vi "Initialize Hardware References.vi"(8 "error in (no error)":errorcluster, 11 "Hardware Resources in":T1={"DAQmx Channel 1"="", "DAQmx Channel 2"="", "DAQmx Channel 3"="", "Channel 1 Name"="Battery Voltage", "Channel 2 Name"="Battery Current", "Channel 3 Name"="Brake torque", "Input Config Channel 1"=-1, "Input Config Channel 2"=-1, "Input Config Channel 3"=-1, "Offset Channel 1"=0.0, "Offset Channel 2"=0.0, "Offset Channel 3"=0.0, "Scale Channel 1"=0.0, "Scale Channel 2"=0.0, "Scale Channel 3"=0.0, "Sample time"=50, "Samples per second"=1000.0, "Sample mode"=0, "Samples per channel"=0, "DAQmx AI Task"="", "DAQmx Channel 4"="", "Channel 3 Name 2"="", "Input Config Channel 4"=-1, "Offset Channel 4"=0.0, "Scale Channel 4"=0.0} {"Input Config Channel 4" items=["Default"=-1, "RSE"=10083, "NRSE"=10078, "Differential"=10106, "Pseudodifferential"=12529]; "Input Config Channel 3" items=["Default"=-1, "RSE"=10083, "NRSE"=10078, "Differential"=10106, "Pseudodifferential"=12529]; "Input Config Channel 2" items=["Default"=-1, "RSE"=10083, "NRSE"=10078, "Differential"=10106, "Pseudodifferential"=12529]; "Input Config Channel 1" items=["Default"=-1, "RSE"=10083, "NRSE"=10078, "Differential"=10106, "Pseudodifferential"=12529]; "Sample mode" items=["Hardware Timed Single Point"=12522, "Finite Samples"=10178, "Continuous Samples"=10123]}) -> (0 "error out":errorcluster, 3 "Hardware Resources out":T1={"DAQmx Channel 1"="", "DAQmx Channel 2"="", "DAQmx Channel 3"="", "Channel 1 Name"="Battery Voltage", "Channel 2 Name"="Battery Current", "Channel 3 Name"="Brake torque", "Input Config Channel 1"=-1, "Input Config Channel 2"=-1, "Input Config Channel 3"=-1, "Offset Channel 1"=0.0, "Offset Channel 2"=0.0, "Offset Channel 3"=0.0, "Scale Channel 1"=0.0, "Scale Channel 2"=0.0, "Scale Channel 3"=0.0, "Sample time"=50, "Samples per second"=1000.0, "Sample mode"=0, "Samples per channel"=0, "DAQmx AI Task"="", "DAQmx Channel 4"="", "Channel 3 Name 2"="", "Input Config Channel 4"=-1, "Offset Channel 4"=0.0, "Scale Channel 4"=0.0} {"Input Config Channel 4" items=["Default"=-1, "RSE"=10083, "NRSE"=10078, "Differential"=10106, "Pseudodifferential"=12529]; "Input Config Channel 3" items=["Default"=-1, "RSE"=10083, "NRSE"=10078, "Differential"=10106, "Pseudodifferential"=12529]; "Input Config Channel 2" items=["Default"=-1, "RSE"=10083, "NRSE"=10078, "Differential"=10106, "Pseudodifferential"=12529]; "Input Config Channel 1" items=["Default"=-1, "RSE"=10083, "NRSE"=10078, "Differential"=10106, "Pseudodifferential"=12529]; "Sample mode" items=["Hardware Timed Single Point"=12522, "Finite Samples"=10178, "Continuous Samples"=10123]})   [LabVIEW 2018, in "Acquisition.lvlib"]
doc: "Initialize the hardware references."
uses:
  Acquisition.lvlib
  Hardware Configuration.ctl
  <vilib>/DAQmx/create/channels.llb/DAQmx Create Channel (AI-Voltage-Basic).vi
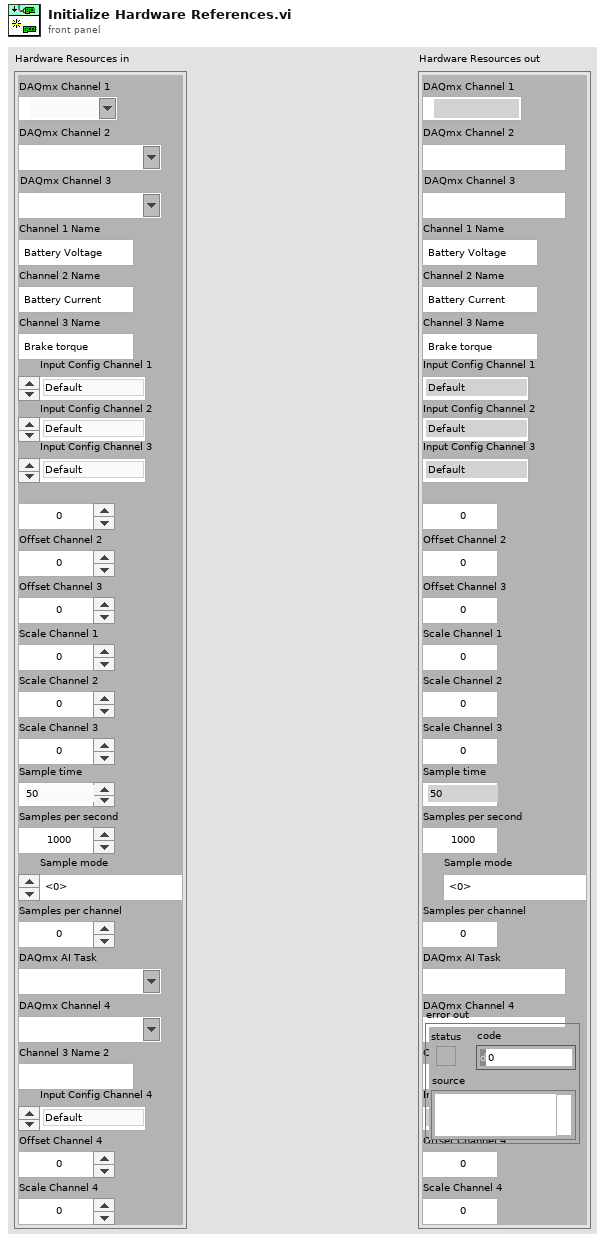
[diagram p1: front panel]
types:
  T1 = typedef "Acquisition.lvlib/Hardware Configuration.ctl" = cluster{"DAQmx Channel 1":tag, "DAQmx Channel 2":tag, "DAQmx Channel 3":tag, "Channel 1 Name":string, "Channel 2 Name":string, "Channel 3 Name":string, "Input Config Channel 1":i32, "Input Config Channel 2":i32, "Input Config Channel 3":i32, "Offset Channel 1":dbl, "Offset Channel 2":dbl, "Offset Channel 3":dbl, "Scale Channel 1":dbl, "Scale Channel 2":dbl, "Scale Channel 3":dbl, "Sample time":u32, "Samples per second":dbl, "Sample mode":u16, "Samples per channel":i32, "DAQmx AI Task":refnum<k21>, "DAQmx Channel 4":tag, "Channel 3 Name 2":string, "Input Config Channel 4":i32, "Offset Channel 4":dbl, "Scale Channel 4":dbl}
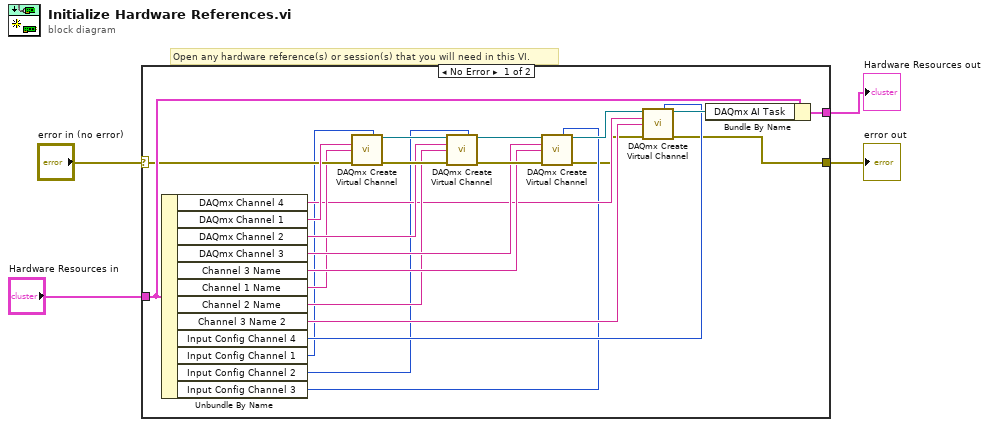
[diagram p0: block diagram]
diagram:
  # "Open any hardware reference(s) or session(s) that you will need in this VI."
  n1 = case shown="No Error" "error in (no error)" {
    selector: "error in (no error)" -> [w24 w28]
    tunnel: [w5 w28] -> w3
    tunnel: "Hardware Resources in" -> [w26 w29]
    tunnel: [w27 w29] -> w1
    frame No Error {
      n2 = Unbundle By Name(w26) -> ("DAQmx Channel 4"=w13:tag, "DAQmx Channel 1"=w25:tag, "DAQmx Channel 2"=w19:tag, "DAQmx Channel 3"=w18:tag, "Channel 3 Name"=w17:string, "Channel 1 Name"=w15:string, "Channel 2 Name"=w16:string, "Channel 3 Name 2"=w14:string, "Input Config Channel 4"=w10:i32, "Input Config Channel 1"=w7:i32, "Input Config Channel 2"=w8:i32, "Input Config Channel 3"=w9:i32)
      n3 = call-poly <vilib>:"DAQmx Create Virtual Channel.vi"("input terminal configuration"=w7, "physical channels"=w25, "name to assign"=w15, "error in"=w24) -> ("task out"=w21:refnum<k21>, "error out"=w23:errorcluster)  [unwired: 10 in]
      n4 = call-poly <vilib>:"DAQmx Create Virtual Channel.vi"("task in"=w21, "input terminal configuration"=w8, "physical channels"=w19, "name to assign"=w16, "error in"=w23) -> ("task out"=w20:refnum<k21>, "error out"=w22:errorcluster)  [unwired: 9 in]
      n5 = call-poly <vilib>:"DAQmx Create Virtual Channel.vi"("task in"=w20, "input terminal configuration"=w9, "physical channels"=w18, "name to assign"=w17, "error in"=w22) -> ("task out"=w12:refnum<k21>, "error out"=w6:errorcluster)  [unwired: 9 in]
      n6 = call-poly <vilib>:"DAQmx Create Virtual Channel.vi"("task in"=w12, "input terminal configuration"=w10, "physical channels"=w13, "name to assign"=w14, "error in"=w6) -> ("task out"=w11:refnum<k21>, "error out"=w5:errorcluster)  [unwired: 9 in]
      n7 = Bundle By Name(cluster=w26, "DAQmx AI Task"=w11) -> (w27:T1)
    }
    frame Error {
    }
  }
  "Hardware Resources out" <- w1
  "error out" <- w3
